vi "get_Gain.vi"(8 "error in (no error)":errorcluster, 11 "GenericDetector in":refnum<class "GenericDetector.lvclass">) -> (0 "error out":errorcluster, 2 "Gain":dbl, 3 "GenericDetector out":refnum<class "GenericDetector.lvclass">)   [LabVIEW 2010, in "GenericDetector.lvclass"]
uses:
  GenericDetector.lvclass
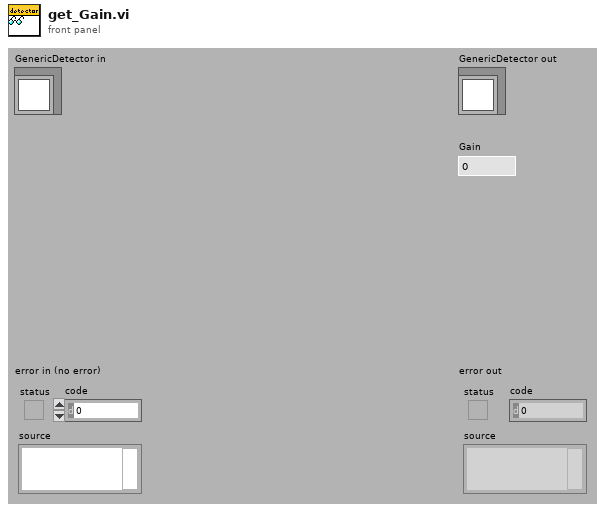
[diagram p1: front panel]
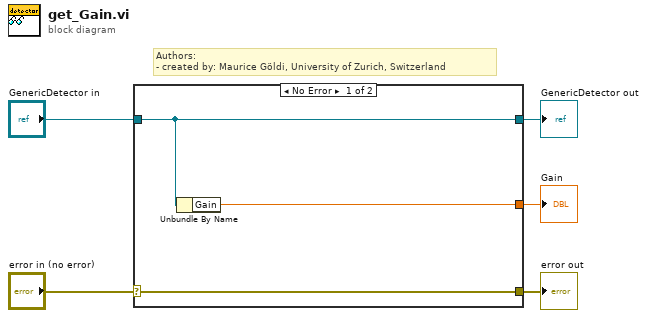
[diagram p0: block diagram]
diagram:
  # "Authors: \n- created by: Maurice Göldi, University of Zurich, Switzerland"
  n1 = case shown="No Error" "error in (no error)" {
    selector: "error in (no error)" -> [w8 w9]
    tunnel: [w8 w9] -> w4
    tunnel: [w7 w10] -> w2
    tunnel: "GenericDetector in" -> [w7 w10]
    tunnel: [w6 _] -> w1
    frame No Error {
      n2 = Unbundle By Name(w7) -> ("Gain"=w6:dbl)
    }
    frame Error {
    }
  }
  "error out" <- w4
  "GenericDetector out" <- w2
  "Gain" <- w1
